vi "Check if configuration files exist.vi"(8 "error in (no error)":errorcluster, 11 "TomoBase in":refnum<class "Tomo.lvclass">) -> (0 "error out":errorcluster, 2 "configuration file exists?":bool, 3 "TomoBase out":refnum<class "Tomo.lvclass">)   [LabVIEW 2012, in "Tomo.lvclass"]
doc: "Checks whether all required configuration files for the component exist."
uses:
  Tomo.lvclass
  <vilib>/Distrio/Murmex/Murmex/Murmex.lvclass
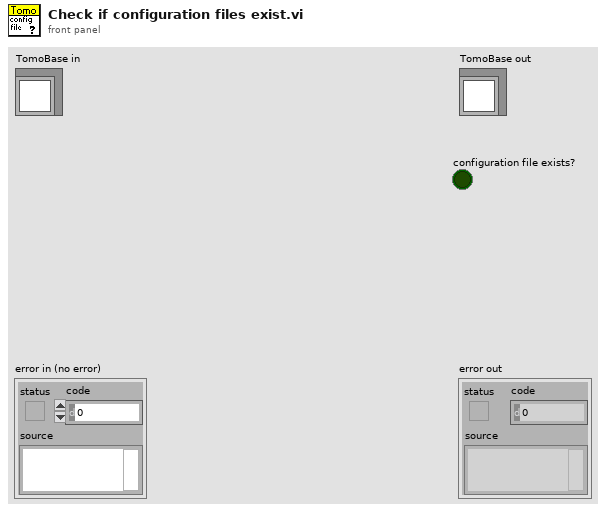
[diagram p1: front panel]
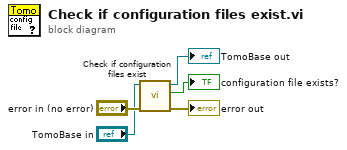
[diagram p0: block diagram]
diagram:
  n1 = call-parent "Check if configuration files exist.vi"("error in (no error)"="error in (no error)", "MurmexBase in"="TomoBase in") -> ("error out"=→"error out":errorcluster, "configuration file exists?"=→"configuration file exists?":bool, "MurmexBase out"=→"TomoBase out":refnum<class "Tomo.lvclass">)  [unwired: 7 in]
